vi "TIO RPC Parse Reply.vi"(11 "Payload":string) -> (2 "Payload":string, 3 "Request ID":u16)   [LabVIEW 2019]
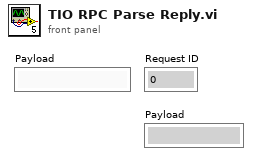
[diagram p1: front panel]
types:
  T1 = enum16{"big-endian, network order", "native, host order", "little-endian"}
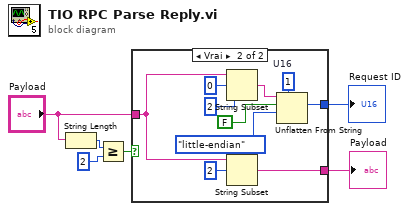
[diagram p0: block diagram]
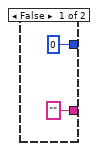
[diagram p2: hidden frame]
diagram:
  n1 = String Length(string="Payload") -> (length=w2:i32)
  n2 = Greater Or Equal?(x=w2, y=2) -> (x >= y?=w1:bool)
  n3 = case shown="Vrai" w1 {
    tunnel: ["" ("Payload") w18] -> w6
    tunnel: [u16 0 ("U16") w11] -> w5
    tunnel: "Payload" -> [_ w10]
    frame False {
    }
    frame True {
      w15 = u16 1  # U16
      n4 = String Subset(string=w10, offset (0)=0, length (rest)=2 ("length (rest)")) -> (substring=w12:string)
      n5 = String Subset(string=w10, offset (0)=2) -> (substring=w18:string)  [unwired: 1 in]
      n6 = Unflatten From String(type=w15, binary string=w12, data includes array or string size? (T)=FALSE, byte order (0:big-endian, network order)=T1."little-endian") -> (value=w11:u16)  [unwired: 1 in, 2 out]
    }
  }
  "Payload" <- w6
  "Request ID" <- w5
